vi "HS_ConvertJPG.vi"(11 "buffer":string) -> (1 "image data":T1, 3 "new picture":picture)   [LabVIEW 2016]
uses:
  <vilib>/picture/picture.llb/imagedata.ctl
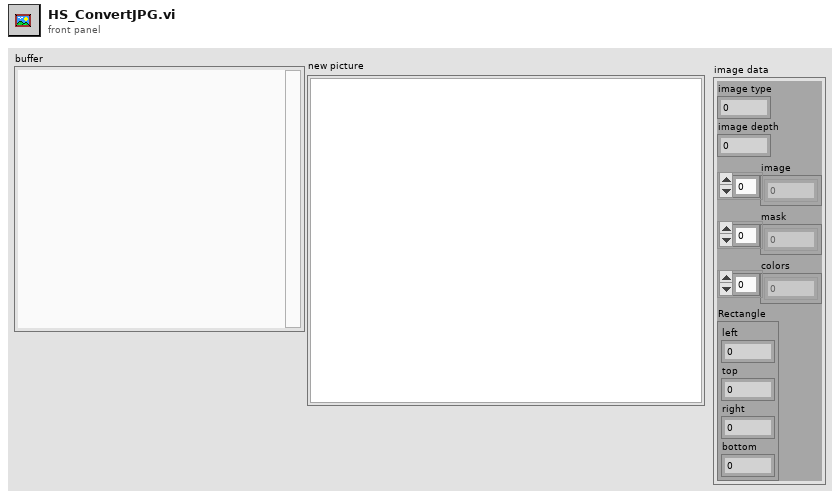
[diagram p1: front panel]
types:
  T1 = typedef "imagedata.ctl" = cluster{"image type":i32, "image depth":i32, "image":u8[], "mask":u8[], "colors":u32[], "Rectangle":cluster{"left":i16, "top":i16, "right":i16, "bottom":i16}}
  T2 = enum16{"big-endian, network order", "native, host order", "little-endian"}
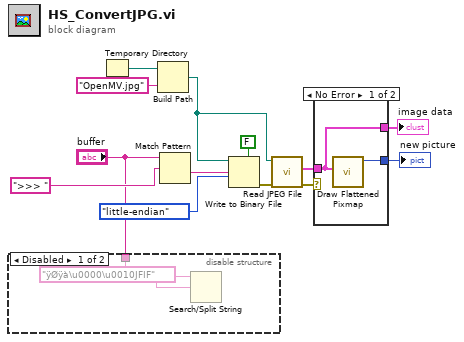
[diagram p0: block diagram]
diagram:
  n1 = disable-structure shown="Disabled" {
    disable-tunnel: "buffer" -> [w14 _]
    frame Disabled {
      n2 = Search/Split String(string=w14, search string/char (-)="ÿØÿà\u0000\u0010JFIF") -> ()  [unwired: 1 in, 3 out]
    }
    frame Enabled {
    }
  }
  n3 = Temporary Directory() -> (w6:path)
  n4 = Build Path(base path=w6, name or relative path="OpenMV.jpg") -> (appended path=w4:path)
  n5 = Match Pattern(string="buffer", regular expression=">>> ") -> (after substring=w1:string)  [unwired: 1 in, 3 out]
  n6 = Write to Binary File(file (use dialog)=w4, data=w1, 5:FALSE ("prepend array or string size? (T)"), 9:T2."little-endian" ("byte order (0:big-endian, network order)")) -> (error out=w11:errorcluster)  [unwired: 2 in, 2 out]
  n7 = call <vilib>:"Read JPEG File.vi"("error in (no error)"=w11, "path to JPEG file"=w4) -> ("error out"=w7:errorcluster, "image data"=w10:T1)  [unwired: 7 in, 1 out]
  n8 = case shown="No Error" w7 {
    tunnel: w10 -> [w16 _]
    tunnel: [w17 _] -> w9
    tunnel: [w16 _] -> w3
    frame No Error {
      n9 = call <vilib>:"Draw Flattened Pixmap.vi"("image data"=w16) -> ("new picture"=w17:picture)  [unwired: 8 in]
    }
    frame Error {
    }
  }
  "new picture" <- w9
  "image data" <- w3
